vi "Humidity Bricklet Test.vi"() -> ()   [LabVIEW 2011]
uses:
  Classes/Device/Type Definitions/Callback Option.ctl
  Classes/IP Connection/IP Connection.lvclass
  Classes/Device/Device.lvclass
  Classes/Humidity Bricklet/Humidity Bricklet.lvclass
panel:
  out "appended array":bool[](array[boolean])
  out "x-y":u32
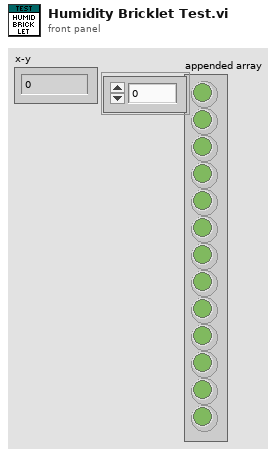
[diagram p1: front panel]
types:
  T1 = typedef "Tinkerforge.lvlib/Device.lvclass/Callback Option.ctl" = enum8{"CB off", "outside range", "inside range", "smaller", "greater"}
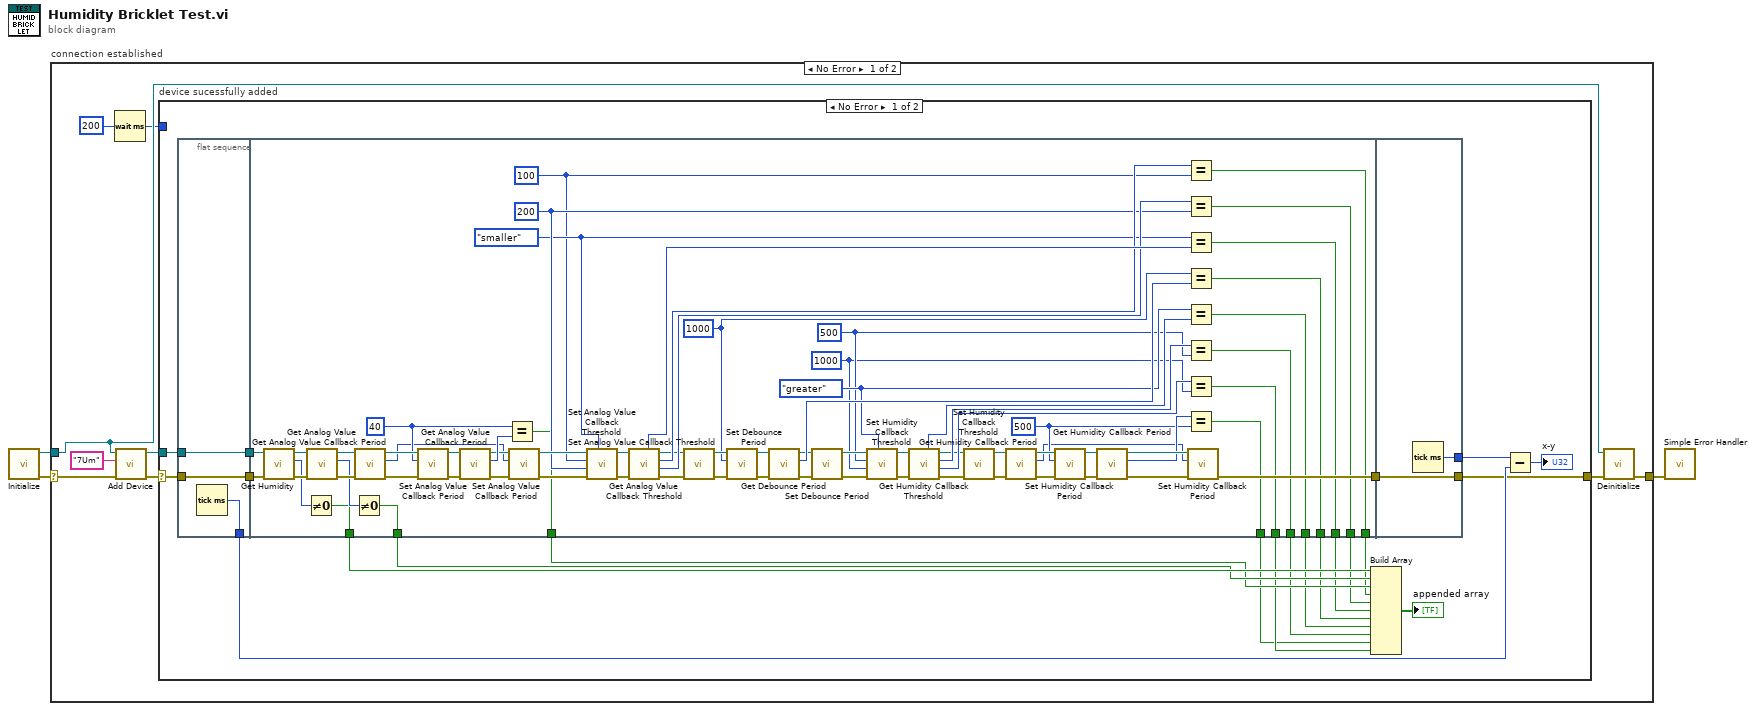
[diagram p0: block diagram]
diagram:
  n1 = call "Initialize.vi"() -> ("error out"=w1:errorcluster, "IP Connection out"=w3:refnum<class "IP Connection.lvclass">)  [unwired: 10 in]
  n2 = case "connection established" shown="No Error" w1 {
    selector: w1 -> [w8 w112]
    tunnel: w3 -> [w12 _]
    tunnel: [w4 w112] -> w2
    frame No Error {
      n3 = Wait (ms)(milliseconds to wait=u32 200) -> (millisecond timer value=w5:u32)
      n4 = call "Add Device.vi"("Error In"=w8, "Device UID"="7Um", "IP Connection"=w12) -> ("Error Out"=w7:errorcluster, "Humidity Bricklet"=w9:refnum<class "Humidity Bricklet.lvclass">)  [unwired: 7 in]
      n5 = case "device sucessfully added" shown="No Error" w7 {
        selector: w7 -> [w33 w111]
        tunnel: [w13 w111] -> w10
        tunnel: w9 -> [w32 _]
        tunnel: w5 -> [_ _]
        frame No Error {
          n6 = flat-sequence {
            tunnel: w32 -> [w35]
            tunnel: w33 -> [w36]
            tunnel: [w36] -> w30
            tunnel: [w35] -> w29
            tunnel: [w34] -> w27
            tunnel: [w48] -> w31
            tunnel: w30 -> [w108]
            tunnel: w29 -> [w107]
            tunnel: [w47] -> w25
            tunnel: [w46] -> w24
            tunnel: [w45] -> w23
            tunnel: [w44] -> w22
            tunnel: [w43] -> w21
            tunnel: [w42] -> w20
            tunnel: [w41] -> w19
            tunnel: [w40] -> w18
            tunnel: [w39] -> w17
            tunnel: [w38] -> w16
            tunnel: [w37] -> w15
            tunnel: [w110] -> w13
            tunnel: w31 -> [w110]
            tunnel: [w109] -> w28
            frame #0 {
              n7 = Tick Count (ms)() -> (millisecond timer value=w34:u32)
            }
            frame #1 {
              w50 = u32 500 ("period (0: off)")
              w62 = i16 1000 ("max")
              w64 = i16 500 ("min")
              w67 = Callback_Option."greater" ("Callback Option (off)")
              w77 = u32 1000 ("debounce (100)")
              w85 = i16 200 ("max")
              w70 = i16 100 ("min")
              w71 = Callback_Option."smaller" ("Callback Option (off)")
              w97 = u32 40
              n8 = call "Get Humidity.vi"("error in (no error)"=w108, "Humidity Bricklet in"=w107) -> ("error out"=w106:errorcluster, "Humidity"=w96:u16, "Humidity Bricklet out"=w105:refnum<class "Humidity Bricklet.lvclass">)  [unwired: 7 in]
              n9 = Not Equal To 0?(x=w96) -> (x != 0?=w47:bool)
              n10 = call "Get Analog Value.vi"("error in (no error)"=w106, "Humidity Bricklet in"=w105) -> ("error out"=w104:errorcluster, "Analog Value"=w95:u16, "Humidity Bricklet out"=w99:refnum<class "Humidity Bricklet.lvclass">)  [unwired: 7 in]
              n11 = Not Equal To 0?(x=w95) -> (x != 0?=w46:bool)
              n12 = call "Get Analog Value Callback Period.vi"("error in (no error)"=w104, "Humidity Bricklet in"=w99) -> ("error out"=w103:errorcluster, "period"=w92:u32, "Humidity Bricklet out"=w100:refnum<class "Humidity Bricklet.lvclass">)  [unwired: 7 in]
              n13 = call "Set Analog Value Callback Period.vi"("error in (no error)"=w103, "period (0: off)"=w97, "Humidity Bricklet in"=w100) -> ("error out"=w102:errorcluster, "Humidity Bricklet out"=w101:refnum<class "Humidity Bricklet.lvclass">)  [unwired: 7 in]
              n14 = call "Get Analog Value Callback Period.vi"("error in (no error)"=w102, "Humidity Bricklet in"=w101) -> ("error out"=w94:errorcluster, "period"=w98:u32, "Humidity Bricklet out"=w93:refnum<class "Humidity Bricklet.lvclass">)  [unwired: 7 in]
              n15 = Equal?(x=w97, y=w98) -> (x = y?=w45:bool)
              n16 = call "Set Analog Value Callback Period.vi"("error in (no error)"=w94, "period (0: off)"=w92, "Humidity Bricklet in"=w93) -> ("error out"=w91:errorcluster, "Humidity Bricklet out"=w89:refnum<class "Humidity Bricklet.lvclass">)  [unwired: 7 in]
              n17 = call "Set Analog Value Callback Threshold.vi"("Callback Option (off)"=w71, "error in (no error)"=w91, "max"=w85, "min"=w70, "Humidity Bricklet in"=w89) -> ("error out"=w90:errorcluster, "Humidity Bricklet out"=w84:refnum<class "Humidity Bricklet.lvclass">)  [unwired: 5 in]
              n18 = call "Get Analog Value Callback Threshold.vi"("error in (no error)"=w90, "Humidity Bricklet in"=w84) -> ("error out"=w83:errorcluster, "max"=w86:i16, "min"=w87:i16, "Humidity Bricklet out"=w82:refnum<class "Humidity Bricklet.lvclass">, "Callback Option"=w88:T1)  [unwired: 5 in]
              n19 = call "Set Analog Value Callback Threshold.vi"("error in (no error)"=w83, "Humidity Bricklet in"=w82) -> ("error out"=w81:errorcluster, "Humidity Bricklet out"=w80:refnum<class "Humidity Bricklet.lvclass">)  [unwired: 8 in]
              n20 = call "Set Debounce Period.vi"("error in (no error)"=w81, "debounce (100)"=w77, "Humidity Bricklet in"=w80) -> ("error out"=w78:errorcluster, "Humidity Bricklet out"=w79:refnum<class "Humidity Bricklet.lvclass">)  [unwired: 7 in]
              n21 = call "Get Debounce Period.vi"("error in (no error)"=w78, "Humidity Bricklet in"=w79) -> ("error out"=w75:errorcluster, "debounce"=w76:u32, "Humidity Bricklet out"=w74:refnum<class "Humidity Bricklet.lvclass">)  [unwired: 7 in]
              n22 = call "Set Debounce Period.vi"("error in (no error)"=w75, "Humidity Bricklet in"=w74) -> ("error out"=w73:errorcluster, "Humidity Bricklet out"=w72:refnum<class "Humidity Bricklet.lvclass">)  [unwired: 8 in]
              n23 = call "Set Humidity Callback Threshold.vi"("Callback Option (off)"=w67, "error in (no error)"=w73, "max"=w62, "min"=w64, "Humidity Bricklet in"=w72) -> ("error out"=w69:errorcluster, "Humidity Bricklet out"=w68:refnum<class "Humidity Bricklet.lvclass">)  [unwired: 5 in]
              n24 = call "Get Humidity Callback Threshold.vi"("error in (no error)"=w69, "Humidity Bricklet in"=w68) -> ("error out"=w61:errorcluster, "max"=w63:i16, "min"=w65:i16, "Humidity Bricklet out"=w60:refnum<class "Humidity Bricklet.lvclass">, "Callback Option"=w66:T1)  [unwired: 5 in]
              n25 = call "Set Humidity Callback Threshold.vi"("error in (no error)"=w61, "Humidity Bricklet in"=w60) -> ("error out"=w59:errorcluster, "Humidity Bricklet out"=w58:refnum<class "Humidity Bricklet.lvclass">)  [unwired: 8 in]
              n26 = call "Get Humidity Callback Period.vi"("error in (no error)"=w59, "Humidity Bricklet in"=w58) -> ("error out"=w57:errorcluster, "period"=w49:u32, "Humidity Bricklet out"=w56:refnum<class "Humidity Bricklet.lvclass">)  [unwired: 7 in]
              n27 = call "Set Humidity Callback Period.vi"("error in (no error)"=w57, "period (0: off)"=w50, "Humidity Bricklet in"=w56) -> ("error out"=w54:errorcluster, "Humidity Bricklet out"=w53:refnum<class "Humidity Bricklet.lvclass">)  [unwired: 7 in]
              n28 = call "Get Humidity Callback Period.vi"("error in (no error)"=w54, "Humidity Bricklet in"=w53) -> ("error out"=w52:errorcluster, "period"=w51:u32, "Humidity Bricklet out"=w55:refnum<class "Humidity Bricklet.lvclass">)  [unwired: 7 in]
              n29 = Equal?(x=w87, y=w70) -> (x = y?=w44:bool)
              n30 = Equal?(x=w86, y=w85) -> (x = y?=w43:bool)
              n31 = Equal?(x=w71, y=w88) -> (x = y?=w42:bool)
              n32 = Equal?(x=w77, y=w76) -> (x = y?=w41:bool)
              n33 = Equal?(x=w67, y=w66) -> (x = y?=w40:bool)
              n34 = Equal?(x=w65, y=w64) -> (x = y?=w39:bool)
              n35 = Equal?(x=w63, y=w62) -> (x = y?=w38:bool)
              n36 = Equal?(x=w51, y=w50) -> (x = y?=w37:bool)
              n37 = call "Set Humidity Callback Period.vi"("error in (no error)"=w52, "period (0: off)"=w49, "Humidity Bricklet in"=w55) -> ("error out"=w48:errorcluster)  [unwired: 7 in, 1 out]
            }
            frame #2 {
              n38 = Tick Count (ms)() -> (millisecond timer value=w109:u32)
            }
          }
          n39 = Build Array(w25, w24, w23, w22, w21, w20, w19, w18, w17, w15, w16) -> (→"appended array":bool[])
          n40 = Subtract(x=w28, y=w27) -> (x-y=→"x-y":u32)
        }
        frame Error {
        }
      }
      n41 = call "Deinitialize.vi"("error in (no error)"=w10, "IP Connection in"=w12) -> ("error out"=w4:errorcluster)  [unwired: 9 in]
    }
    frame Error {
    }
  }
  n42 = call <vilib>:"Simple Error Handler.vi"("error in (no error)"=w2) -> ()  [unwired: 4 in, 5 out]
